vi "OCT Processing 2ch functional global.vi"(0 "Data Format":T3, 1 "State":T4, 5 "Linear?":bool, 7 "Real Time":bool=TRUE, 9 "Input Parameters":T2={"Points Per A-Scan"=0, "A-Scans per B-Scan"=0, "Voltage Range"=4.0, "Card Resolution (bits)"=16}, 11 "error in (no error)":errorcluster, 12 "Background":i32[](array[numeric]), 13 "Resample Array":i32[](array[numeric])) -> (3 "Time Out":bool, 4 "Processed OCT Data":T1, 10 "queue out":refnum<queue>, 14 "# elements in queue":i32, 15 "error out":errorcluster)   [LabVIEW 2014]
doc: "Functional global for processing OCT data. The data can either be 1 channel, 2 channel interleaved (ex. ATS 9462), or 2 channels appended (ATS 660). The output cluster Channel A and Channel B may be a single B-Scan or multople B-Scan stored in an array cluster. Same for the Raw Data Channel A and B."
uses:
  Type Defs/OCT Imaging Parameters Cluster.ctl
  Display Raw Data states.ctl
  processing_states.ctl
  Type Defs/OCT DAQ Channel Data Type.ctl
  Type Defs/Processed OCT Data.ctl
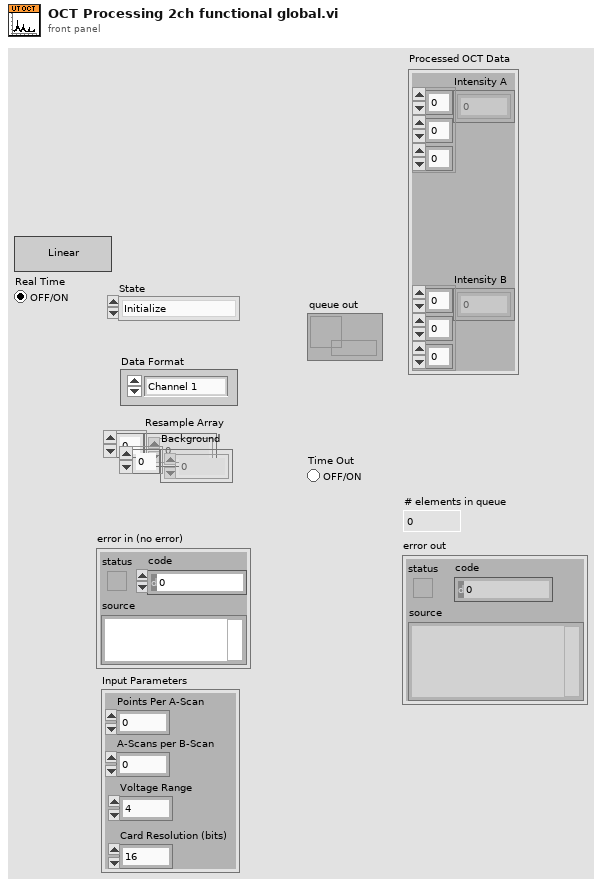
[diagram p1: front panel]
types:
  T1 = typedef "Processed OCT Data.ctl" = cluster{"Intensity A":sgl[][][], "Intensity B":sgl[][][]}
  T2 = typedef "OCT Imaging Parameters Cluster.ctl" = cluster{"Points Per A-Scan":i32, "A-Scans per B-Scan":i32, "Voltage Range":sgl, "Card Resolution (bits)":u16}
  T3 = typedef "OCT DAQ Channel Data Type.ctl" = enum16{"Channel 1", "Channel 2", "Channel 1 and 2"}
  T4 = typedef "processing_states.ctl" = enum16{"Initialize", "Set Background", "Update Imaging Parameters", "Get Queue", "Process Data", "Get Size", "Flush Data", "Set Reample Array", "Get Last Processed BScan", "Shutdown"}
  T5 = typedef "Display Raw Data states.ctl" = enum16{"Add Raw", "Add Processed", "Show"}
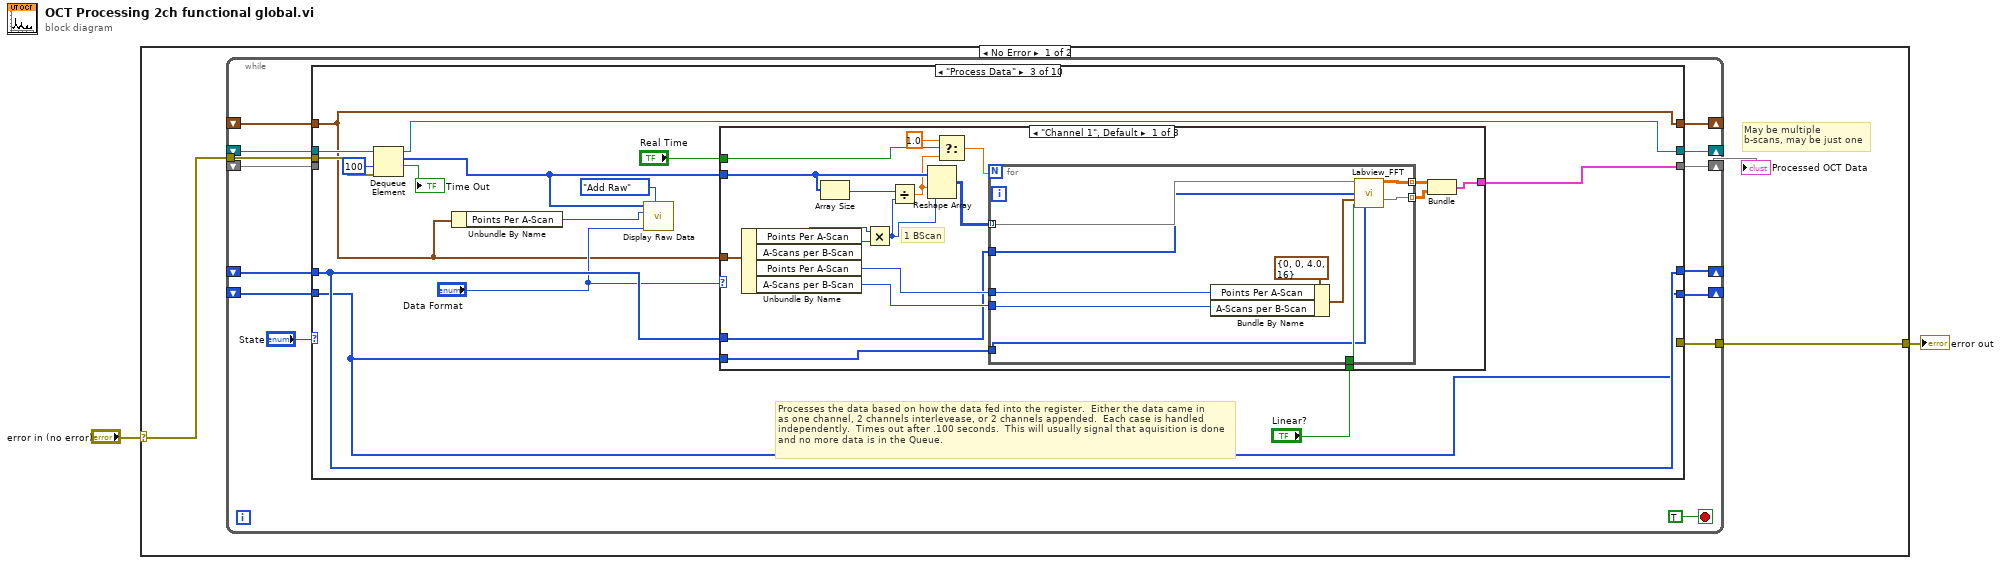
[diagram p0: block diagram]
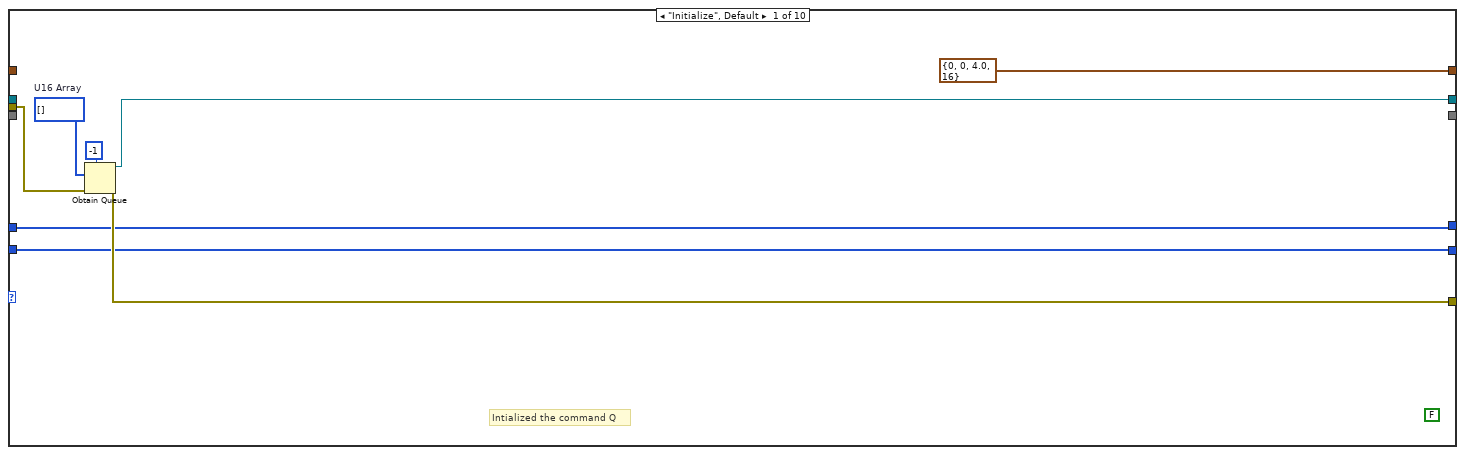
[diagram p2: hidden frame]
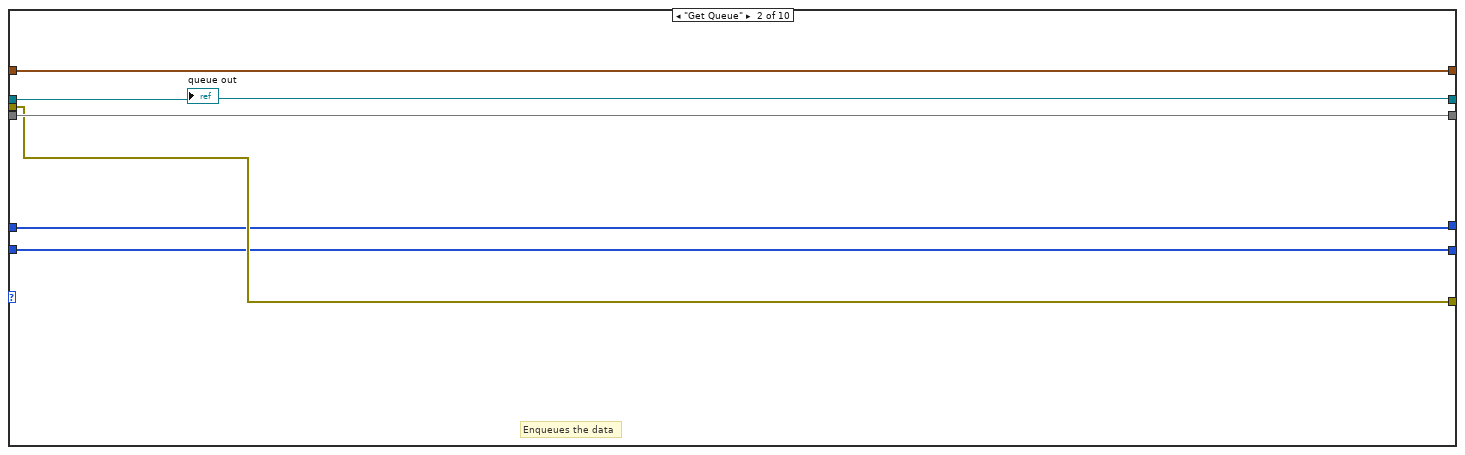
[diagram p3: hidden frame]
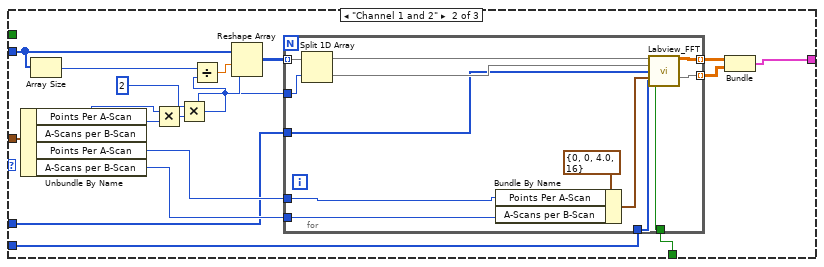
[diagram p4: hidden frame]
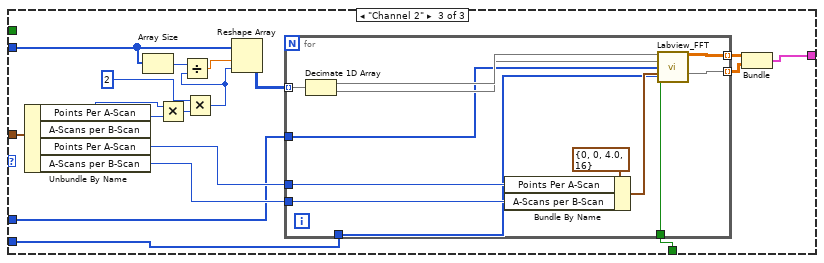
[diagram p5: hidden frame]
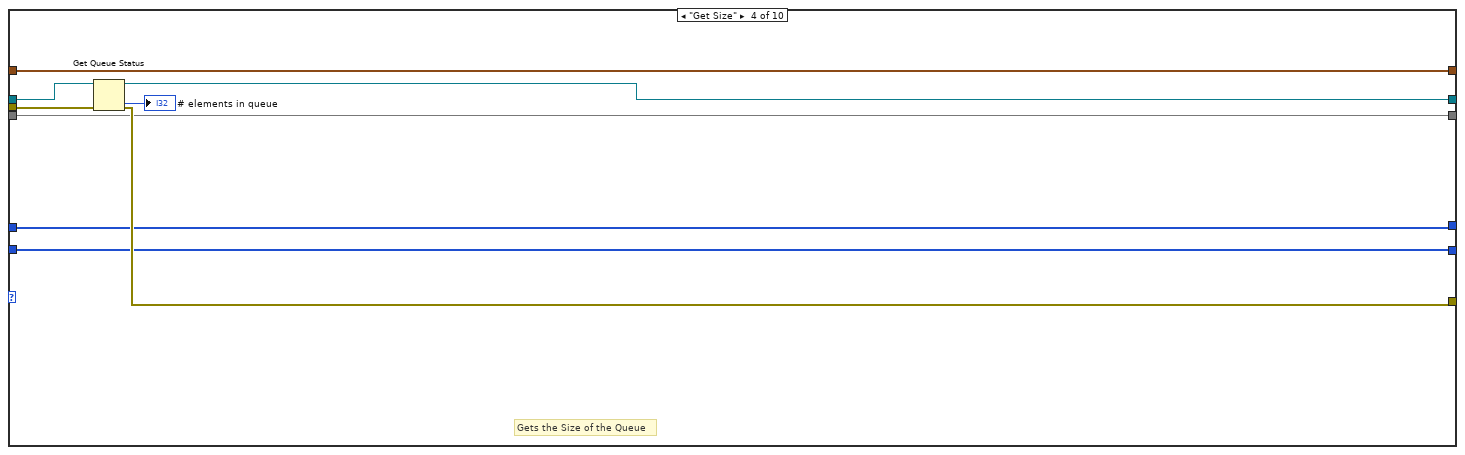
[diagram p6: hidden frame]
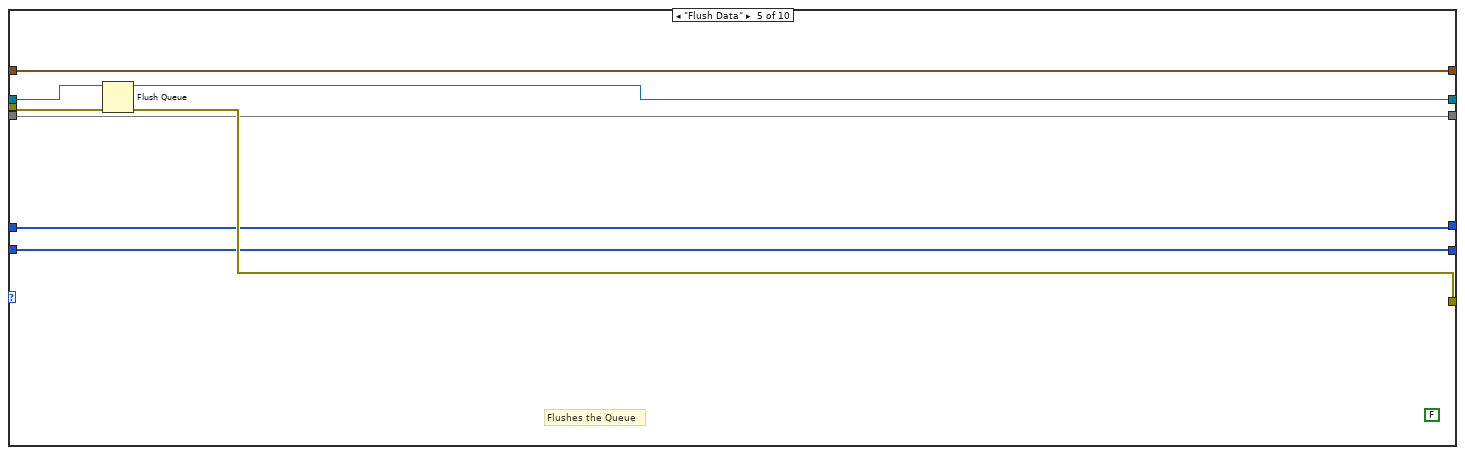
[diagram p7: hidden frame]
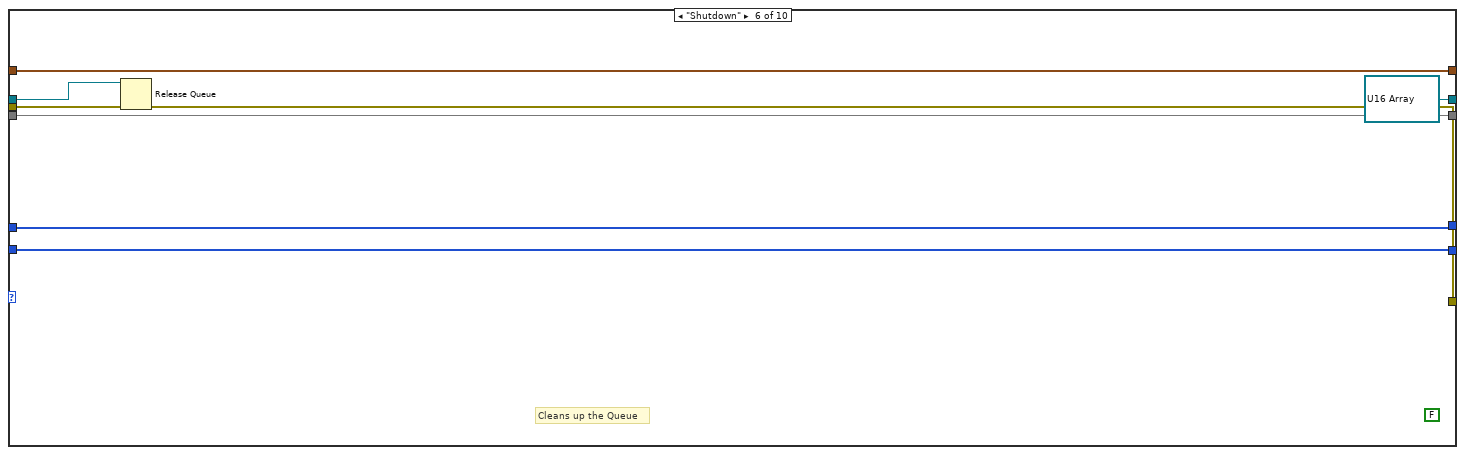
[diagram p8: hidden frame]
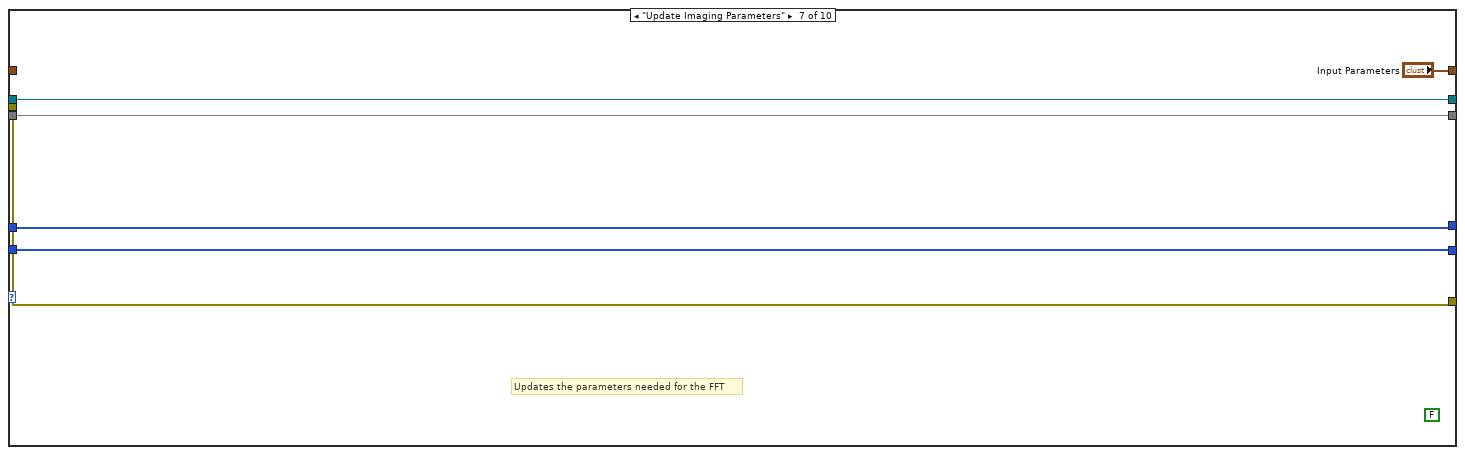
[diagram p9: hidden frame]
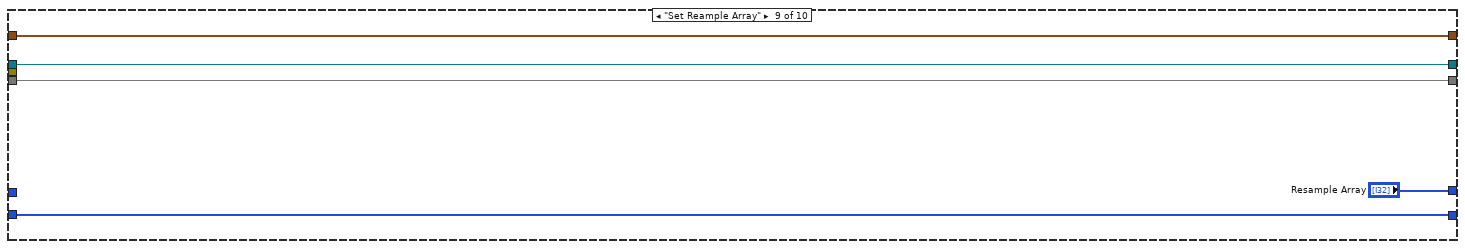
[diagram p11: hidden frame]
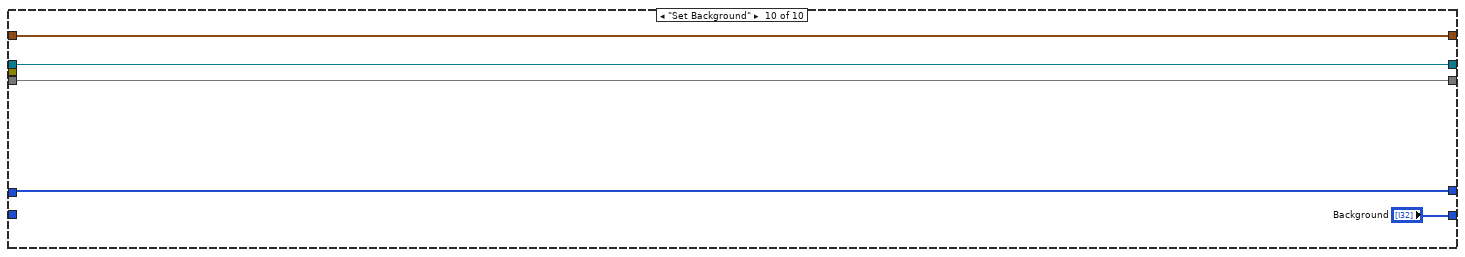
[diagram p12: hidden frame]
diagram:
  n1 = case shown="No Error" "error in (no error)" {
    selector: "error in (no error)" -> [w5 w185]
    tunnel: [w4 w185] -> w1
    frame No Error {
      # "May be multiple\nb-scans, may be just one"
      n2 = while {
        shift-right: [w12] -> _
        shift-left: _ -> [w17]
        tunnel: w5 -> [w18]
        tunnel: [w16] -> w4
        shift-right: [w15] -> _
        shift-left: _ -> [w13]
        shift-right: [w11] -> w3
        shift-left: _ -> [w10]
        shift-right: [w9] -> _
        shift-left: _ -> [w8]
        shift-right: [w6] -> _
        shift-left: _ -> [w7]
        stop <- TRUE stop-if-true
        n3 = case shown="\"Process Data\"" "State" {
          tunnel: [w26 w30 w47 w143 w152 refnum<queue> refnum ("queue out") w169 w174 w176 w182] -> w12
          tunnel: w18 -> [w27 w31 w46 w146 w154 w161 w168 _ _ _]
          tunnel: w17 -> [_ w30 w48 w147 w155 w163 w169 w174 w176 w182]
          tunnel: [w25 w31 _ w144 w153 w160 w168 _ _ _] -> w16
          tunnel: [T2 {"Points Per A-Scan"=0, "A-Scans per B-Scan"=0, "Voltage Range"=4.0, "Card Resolution (bits)"=16} ("Input Parameters") w33 w34 w142 w151 w162 "Input Parameters" w173 w177 w183] -> w15
          tunnel: w13 -> [_ w33 w34 w142 w151 w162 _ w173 w177 w183]
          tunnel: [_ w32 w45 w141 w150 w159 w167 w172 w179 w184] -> w11
          tunnel: w10 -> [_ w32 _ w141 w150 w159 w167 w172 w179 w184]
          tunnel: [w21 w29 w42 w140 w149 w157 w165 w171 "Resample Array" w181] -> w9
          tunnel: w8 -> [w21 w29 w42 w140 w149 w157 w165 w171 _ w181]
          tunnel: w7 -> [w20 w28 w40 w139 w148 w156 w164 w170 w175 _]
          tunnel: [w20 w28 w40 w139 w148 w156 w164 w170 w175 "Background"] -> w6
          frame "Initialize", Default {
            w22 = u16[] []  # U16 Array
            (unwired) FALSE ("timed out?")
            # "Intialized the command Q"
            n4 = Obtain Queue(max queue size (-1, unlimited)=-1, element data type=w22, error in (no error)=w27) -> (queue out=w26:refnum<queue>, error out=w25:errorcluster)  [unwired: 2 in, 1 out]
          }
          frame "Get Queue" {
            # "Enqueues the data"
            "queue out" <- w30
          }
          frame "Process Data" {
            # "Processes the data based on how the data fed into the register.  Either the data came in\nas one channel, 2 channels interlevease, or 2 channels appended.  Each case is handled\nindependently.  Times out after .100 seconds.  This will usually signal that aquisition is done\nand no more data is in the Queue."
            n5 = Dequeue Element(queue=w48, timeout in ms (-1)=100, error in (no error)=w46) -> (queue out=w47:refnum<queue>, element=w37:u16[], timed out?=→"Time Out":bool)  [unwired: 1 out]
            n6 = Unbundle By Name(w34) -> ("Points Per A-Scan"=w35:i32)
            n7 = call "Display Raw Data.vi"("Enum"=Display_Raw_Data_states."Add Raw", "Data Format"="Data Format", "Length"=w35, "Raw Data In"=w37) -> ()  [unwired: 8 in]
            n8 = case shown="\"Channel 1\", Default" "Data Format" {
              tunnel: w37 -> [w58 w93 w124]
              tunnel: w34 -> [w66 w94 w125]
              tunnel: [w62 w88 w119] -> w45
              tunnel: w42 -> [w56 w81 w112]
              tunnel: "Linear?" -> [w55 w80 w111]
              tunnel: w40 -> [w54 w79 w110]
              tunnel: "Real Time" -> [w52 _ _]
              frame "Channel 1", Default {
                # "1 BScan"
                n9 = Unbundle By Name(w66) -> ("Points Per A-Scan"=w61:i32, "A-Scans per B-Scan"=w60:i32, "Points Per A-Scan"=w65:i32, "A-Scans per B-Scan"=w64:i32)
                n10 = Array Size(array=w58) -> (size(s)=w67:i32)
                n11 = Multiply(x=w61, y=w60) -> (x*y=w59:i32)
                n12 = Divide(x=w67, y=w59) -> (x/y=w51:dbl)
                n13 = Reshape Array(w58, w51, w59) -> (w57:u16[][])
                n14 = Select(t=1.0, s=w52, f=w51) -> (s? t:f=w49:dbl)
                n15 = for {
                  N: w49 -> [_]
                  tunnel: w57 -> [w72] mode=indexing
                  tunnel: w65 -> [w71]
                  tunnel: w64 -> [w75]
                  tunnel: [w74] -> w63 mode=indexing
                  tunnel: [w73] -> w53 mode=indexing
                  tunnel: w56 -> [w70]
                  tunnel: w55 -> [w69]
                  tunnel: w54 -> [w68]
                  n16 = Bundle By Name(cluster=T2 {"Points Per A-Scan"=0, "A-Scans per B-Scan"=0, "Voltage Range"=4.0, "Card Resolution (bits)"=16} ("input cluster"), "Points Per A-Scan"=w71, "A-Scans per B-Scan"=w75) -> (w76:T2)
                  n17 = call "Labview_FFT.vi"("Channel A"=w72, "Bits"=w70, 9:w76, 11:w69, 12:w68) -> ("Int B-Scan Channel A"=w74:sgl[][], 10:w73)  [unwired: 9 in]
                }
                n18 = Bundle("Int B-Scan Channel A"=w63, w53) -> (w62:cluster{"Int B-Scan Channel A":sgl[][][], void})  [unwired: 1 in]
              }
              frame "Channel 1 and 2" {
                n19 = Unbundle By Name(w94) -> ("Points Per A-Scan"=w87:i32, "A-Scans per B-Scan"=w86:i32, "Points Per A-Scan"=w91:i32, "A-Scans per B-Scan"=w90:i32)
                n20 = Array Size(array=w93) -> (size(s)=w95:i32)
                n21 = Multiply(x=w87, y=w86) -> (x*y=w82:i32)
                n22 = Multiply(x=2 ("y"), y=w82) -> (x*y=w83:i32)
                n23 = Divide(x=w95, y=w83) -> (x/y=w84:dbl)
                n24 = Reshape Array(w93, w84, w83) -> (w92:u16[][])
                n25 = for {
                  tunnel: w92 -> [w108] mode=indexing
                  tunnel: w91 -> [w101]
                  tunnel: w90 -> [w105]
                  tunnel: [w104] -> w89 mode=indexing
                  tunnel: [w103] -> w78 mode=indexing
                  tunnel: w82 -> [w102]
                  tunnel: w81 -> [w98]
                  tunnel: w80 -> [w97]
                  tunnel: w79 -> [w96]
                  n26 = Split 1D Array(array=w108, index=w102) -> (first subarray=w100:u16[], second subarray=w99:u16[])
                  n27 = Bundle By Name(cluster=T2 {"Points Per A-Scan"=0, "A-Scans per B-Scan"=0, "Voltage Range"=4.0, "Card Resolution (bits)"=16} ("input cluster"), "Points Per A-Scan"=w101, "A-Scans per B-Scan"=w105) -> (w106:T2)
                  n28 = call "Labview_FFT.vi"("Channel A"=w100, "Range"=w99, "Bits"=w98, 9:w106, 11:w97, 12:w96) -> ("Int B-Scan Channel A"=w104:sgl[][], 10:w103)  [unwired: 8 in]
                }
                n29 = Bundle("Int B-Scan Channel A"=w89, w78) -> (w88:cluster{"Int B-Scan Channel A":sgl[][][], void})  [unwired: 1 in]
              }
              frame "Channel 2" {
                n30 = Unbundle By Name(w125) -> ("Points Per A-Scan"=w118:i32, "A-Scans per B-Scan"=w117:i32, "Points Per A-Scan"=w122:i32, "A-Scans per B-Scan"=w121:i32)
                n31 = Array Size(array=w124) -> (size(s)=w126:i32)
                n32 = Multiply(x=w118, y=w117) -> (x*y=w116:i32)
                n33 = Multiply(x=2, y=w116) -> (x*y=w113:i32)
                n34 = Divide(x=w126, y=w113) -> (x/y=w114:dbl)
                n35 = Reshape Array(w124, w114, w113) -> (w123:u16[][])
                n36 = for {
                  tunnel: w123 -> [w138] mode=indexing
                  tunnel: w122 -> [w132]
                  tunnel: w121 -> [w136]
                  tunnel: [w134] -> w120 mode=indexing
                  tunnel: [w133] -> w109 mode=indexing
                  tunnel: w112 -> [w129]
                  tunnel: w111 -> [w128]
                  tunnel: w110 -> [w127]
                  n37 = Decimate 1D Array(w138) -> (w131:u16[], w130:u16[])
                  n38 = Bundle By Name(cluster=T2 {"Points Per A-Scan"=0, "A-Scans per B-Scan"=0, "Voltage Range"=4.0, "Card Resolution (bits)"=16} ("input cluster"), "Points Per A-Scan"=w132, "A-Scans per B-Scan"=w136) -> (w135:T2)
                  n39 = call "Labview_FFT.vi"("Channel A"=w131, "Range"=w130, "Bits"=w129, 9:w135, 11:w128, 12:w127) -> ("Int B-Scan Channel A"=w134:sgl[][], 10:w133)  [unwired: 8 in]
                }
                n40 = Bundle("Int B-Scan Channel A"=w120, w109) -> (w119:cluster{"Int B-Scan Channel A":sgl[][][], void})  [unwired: 1 in]
              }
            }
          }
          frame "Get Size" {
            # "Gets the Size of the Queue"
            n41 = Get Queue Status(queue=w147, error in (no error)=w146) -> (queue out=w143:refnum<queue>, error out=w144:errorcluster, # elements in queue=→"# elements in queue":i32)  [unwired: 1 in, 5 out]
          }
          frame "Flush Data" {
            (unwired) FALSE ("timed out?")
            # "Flushes the Queue"
            n42 = Flush Queue(queue=w155, error in (no error)=w154) -> (queue out=w152:refnum<queue>, error out=w153:errorcluster)  [unwired: 1 out]
          }
          frame "Shutdown" {
            (unwired) FALSE ("timed out?")
            # "Cleans up the Queue"
            n43 = Release Queue(queue=w163, error in (no error)=w161) -> (error out=w160:errorcluster)  [unwired: 1 in, 2 out]
          }
          frame "Update Imaging Parameters" {
            (unwired) FALSE ("timed out?")
            # "Updates the parameters needed for the FFT"
          }
          frame "Get Last Processed BScan" {
            # "Just executes to get the last set of data from the shift register"
          }
          frame "Set Reample Array" {
          }
          frame "Set Background" {
          }
        }
      }
      "Processed OCT Data" <- w3
    }
    frame Error {
    }
  }
  "error out" <- w1
